vi "Teleop.vi"(10 "Match Info":T1={"Autonomous Elapsed Seconds"=0.0, "TeleOp Elapsed Seconds"=0.0, "Disabled Elapsed Seconds"=0.0, "Visited Autonomous"=FALSE, "Visited TeleOp"=FALSE, "Visited Disabled"=FALSE, "Autonomous Settings"={"Autonomous Style"=enum."Independent", "VI Refnum"=refnum}}, 11 "Call Context":T2) -> ()   [LabVIEW 2016]
doc: "This VI is called for each TeleOp packet received from the DS where the robot is not disabled. It is often used to read from the joysticks and update I/O or to update setpoints for timed control loops. It should complete and return within 20 milliseconds or it may miss DS packets."
uses:
  <vilib>/Rock Robotics/WPI/DriverStation/WPI_DriverStationDerivedRobotMode.ctl
  <vilib>/Rock Robotics/WPI/DriverStation/WPI_DriverStationMatch Info.ctl
  <vilib>/Rock Robotics/WPI/Solenoid/WPI_SolenoidValue.ctl
  <vilib>/Rock Robotics/WPI/Utilities/WPI_GetSetVariantRefNum.vi
  <vilib>/Rock Robotics/Network Tables/NT Read Boolean.vi
  <vilib>/Rock Robotics/Network Tables/NT Read Number.vi
  <vilib>/Rock Robotics/WPI/Solenoid/WPI_SolenoidSetEnum.vi
panel:
  in  "Compresseur Limit Time":bool
  in  "Reset":bool
  out "Droit":dbl
  out "Gauche":dbl
  in  "Quand arreter compresseur":dbl
  out "Teleop Time Elipsed":dbl
  out "Sample Slider 0":dbl(slide) scale=0.0..5.0
  out "Sample Boolean 1":bool
  out "Sample Boolean 0":bool
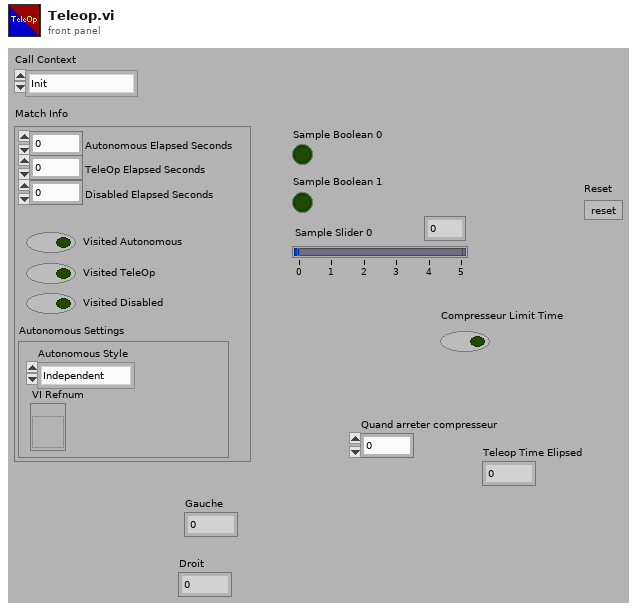
[diagram p1: front panel]
types:
  T1 = typedef "WPI_DriverStationMatch Info.ctl" = cluster{"Autonomous Elapsed Seconds":dbl, "TeleOp Elapsed Seconds":dbl, "Disabled Elapsed Seconds":dbl, "Visited Autonomous":bool, "Visited TeleOp":bool, "Visited Disabled":bool, "Autonomous Settings":cluster{"Autonomous Style":enum16{"Iterative", "Independent"}, "VI Refnum":refnum<vi>}}
  T2 = typedef "WPI_DriverStationDerivedRobotMode.ctl" = enum16{"Init", "Execute", "Stop"}
  T3 = typedef "WPI_JoystickDevRef.ctl" = cluster{"Device":T4}
  T4 = typedef "WPI_JoystickDeviceEnum.ctl" = enum16{"USB 0", "USB 1", "USB 2", "USB 3", "USB 4", "USB 5"}
  T5 = typedef "WPI_EncoderDevRef.ctl" = cluster{"DevStatus":errorcluster, "EncoderIndex":T6, "CounterIndex":T7, "DistancePerCount":dbl, "Decoding Type":T8}
  T6 = typedef "FPGA_EncoderIdx.ctl" = enum8{"Enc 0", "Enc 1", "Enc 2", "Enc 3", "Enc 4", "Enc 5", "Enc 6", "Enc 7", "Invalid"}
  T7 = typedef "FPGA_CounterCtrSystemIndex.ctl" = enum8{"Ctr 0", "Ctr 1", "Ctr 2", "Ctr 3", "Ctr 4", "Ctr 5", "Ctr 6", "Ctr 7", "Invalid"}
  T8 = typedef "WPI_EncoderType.ctl" = enum16{"1x", "2x", "4x"}
  T9 = cluster{"Axes[0]":dbl, "Axes[1]":dbl, "Axes[2]":dbl, "Axes[3]":dbl, "Axes[4]":dbl, "Axes[5]":dbl, "Axes[6]":dbl, "Axes[7]":dbl, "Axes[8]":dbl}
  T10 = cluster{"Buttons[0]":bool, "Buttons[1]":bool, "Buttons[2]":bool, "Buttons[3]":bool, "Buttons[4]":bool, "Buttons[5]":bool, "Buttons[6]":bool, "Buttons[7]":bool, "Buttons[8]":bool}
  T11 = typedef "WPI_RobotDriveDevRef.ctl" = cluster{"DevStatus":errorcluster, "Motors[]":T12[], "Square Inputs":bool, "Max Output":dbl}
  T12 = typedef "WPI_MotorControlDeviceRef.ctl" = cluster{"DeviceStatus":errorcluster, "Type":T13, "PWM":cluster{"PWM Channel":T14, "DeadBand":T15}, "CAN":cluster{"Device Number":u8, "SetOutput VI Ref":variant, "GetOutput VI Ref":variant, "Enable VI Ref":variant, "Disable VI Ref":variant, "Data":variant}, "Invert":bool}
  T13 = typedef "WPI_MotorControlType.ctl" = enum16{"PWM", "CAN"}
  T14 = typedef "FPGA_DIOPWMChannel.ctl" = enum8{"PWM 0", "PWM 1", "PWM 2", "PWM 3", "PWM 4", "PWM 5", "PWM 6", "PWM 7", "PWM 8", "PWM 9", "PWM MXP 0", "PWM MXP 1", "PWM MXP 2", "PWM MXP 3", "PWM MXP 4", "PWM MXP 5", "PWM MXP 6", "PWM MXP 7", "PWM MXP 8", "PWM MXP 9", "Invalid"}
  T15 = typedef "WPI_PWMDeadband.ctl" = cluster{"Name":string, "maxPositivePwm":i32, "minPositivePwm":i32, "centerPwm":i32, "maxNegativePwm":i32, "minNegativePwm":i32, "angularRange":u16}
  T16 = typedef "WPI_SolenoidValue.ctl" = enum16{"Off", "On", "Forward", "Reverse"}
  T17 = typedef "WPI_SolenoidDevRef.ctl" = cluster{"DevStatus":errorcluster, "Pneumatics Control Module":u8, "Forward Solenoid Channel":T18, "Reverse Solenoid Channel":T18}
  T18 = typedef "WPI_SolenoidChannel.ctl" = enum8{"Solenoid 0", "Solenoid 1", "Solenoid 2", "Solenoid 3", "Solenoid 4", "Solenoid 5", "Solenoid 6", "Solenoid 7", "Invalid"}
  T19 = typedef "WPI_CompressorDevRef.ctl" = cluster{"DevStatus":errorcluster, "Pneumatics Control Module":u8}
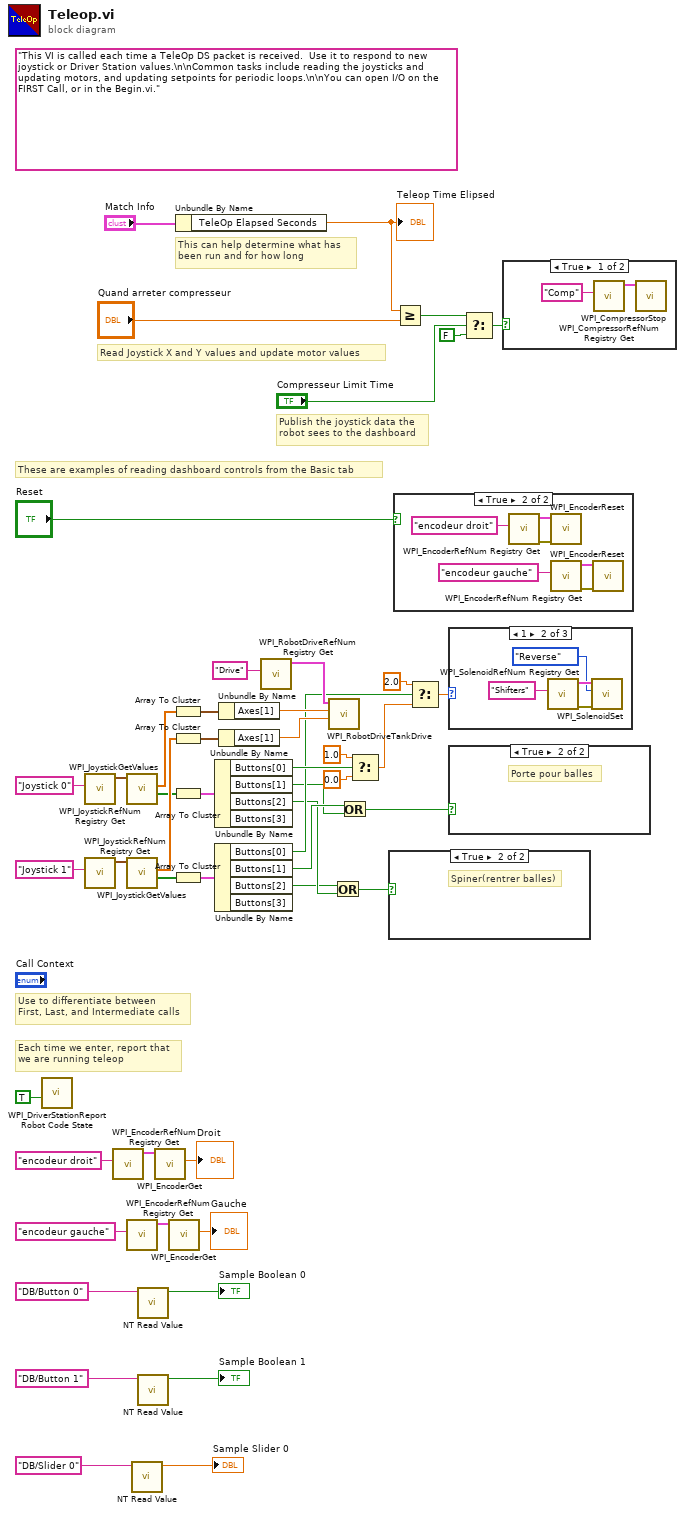
[diagram p0: block diagram]
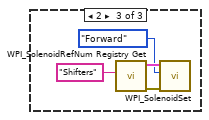
[diagram p7: hidden frame]
diagram:
  (unwired) "This VI is called each time a TeleOp DS packet is received.  Use it to respond to new joystick or Driver Station values.\n\nCommon tasks include reading the joysticks and updating motors, and updating setpoints for periodic loops.\n\nYou can open I/O on the FIRST Call, or in the Begin.vi."
  # "These are examples of reading dashboard controls from the Basic tab"
  # "Publish the joystick data the\nrobot sees to the dashboard"
  # "Each time we enter, report that\nwe are running teleop"
  # "Use to differentiate between\nFirst, Last, and Intermediate calls"
  # "This can help determine what has\nbeen run and for how long"
  # "Read Joystick X and Y values and update motor values"
  n1 = call <vilib>:"WPI_DriverStationReport Robot Code State.vi"("TeleOp"=TRUE ("Autonomous")) -> ()  [unwired: 10 in, 1 out]
  n2 = call <vilib>:"WPI_JoystickRefNum Registry Get.vi"("refnum name"="Joystick 0") -> ("JoystickDevRef"=w48:T3)  [unwired: 1 in, 9 out]
  n3 = call <vilib>:"WPI_JoystickRefNum Registry Get.vi"("refnum name"="Joystick 1") -> ("JoystickDevRef"=w36:T3)  [unwired: 1 in, 9 out]
  n4 = call <vilib>:"WPI_EncoderRefNum Registry Get.vi"("refnum name"="encodeur droit") -> ("EncoderDevRef"=w16:T5)  [unwired: 9 in, 1 out]
  n5 = call <vilib>:"WPI_JoystickGetValues.vi"("JoystickDevRef"=w48) -> ("Buttons"=w27:bool[], "Axes"=w39:dbl[])  [unwired: 6 in, 3 out]
  n6 = call <vilib>:"WPI_JoystickGetValues.vi"("JoystickDevRef"=w36) -> ("Buttons"=w30:bool[], "Axes"=w35:dbl[])  [unwired: 6 in, 3 out]
  n7 = call <vilib>:"WPI_EncoderRefNum Registry Get.vi"("refnum name"="encodeur gauche") -> ("EncoderDevRef"=w17:T5)  [unwired: 9 in, 1 out]
  n8 = call-poly <vilib>:"NT Read Value.vi"("Name"="DB/Slider 0" ("refnum name")) -> ("Numeric"=→"Sample Slider 0":dbl)  [unwired: 9 in, 1 out]
  n9 = call-poly <vilib>:"NT Read Value.vi"("Name"="DB/Button 0" ("refnum name")) -> ("Boolean"=→"Sample Boolean 0":bool)  [unwired: 9 in, 1 out]
  n10 = call-poly <vilib>:"NT Read Value.vi"("Name"="DB/Button 1" ("refnum name")) -> ("Boolean"=→"Sample Boolean 1":bool)  [unwired: 9 in, 1 out]
  n11 = call <vilib>:"WPI_EncoderGet.vi"("EncoderDevRef"=w16) -> ("Distance"=→"Droit":dbl)  [unwired: 5 in, 5 out]
  n12 = call <vilib>:"WPI_EncoderGet.vi"("EncoderDevRef"=w17) -> ("Distance"=→"Gauche":dbl)  [unwired: 5 in, 5 out]
  n13 = Array To Cluster(array=w39) -> (cluster=w38:T9)
  n14 = Array To Cluster(array=w35) -> (cluster=w34:T9)
  n15 = Array To Cluster(array=w27) -> (cluster=w28:T10)
  n16 = Array To Cluster(array=w30) -> (cluster=w29:T10)
  n17 = Unbundle By Name("Match Info") -> ("TeleOp Elapsed Seconds"=w18:dbl)
  "Teleop Time Elipsed" <- w18
  n18 = Unbundle By Name(w28) -> ("Buttons[0]"=w24:bool, "Buttons[1]"=w9:bool, "Buttons[2]"=w8:bool)  [unwired: 1 out]
  n19 = Unbundle By Name(w29) -> ("Buttons[0]"=w22:bool, "Buttons[1]"=w10:bool, "Buttons[2]"=w7:bool)  [unwired: 1 out]
  n20 = Unbundle By Name(w38) -> ("Axes[1]"=w32:dbl)
  n21 = Unbundle By Name(w34) -> ("Axes[1]"=w31:dbl)
  n22 = call <vilib>:"WPI_RobotDriveRefNum Registry Get.vi"("refnum name"="Drive") -> ("RobotDriveDevRef"=w40:T11)  [unwired: 9 in, 1 out]
  n23 = call <vilib>:"WPI_RobotDriveTankDrive.vi"("Right axis value"=w31, "Left axis value"=w32, "RobotDriveDevRef"=w40) -> ()  [unwired: 6 in, 3 out]
  n24 = Or(x=w7, y=w8) -> (x .or. y?=w6:bool)
  n25 = Or(x=w10, y=w9) -> (x .or. y?=w5:bool)
  n26 = Select(t=1.0, s=w24, f=0.0) -> (s? t:f=w26:dbl)
  n27 = case shown="True" w6 {
    frame False {
    }
    frame True {
      # "Spiner(rentrer balles)"
    }
  }
  n28 = case shown="True" "Reset" {
    frame False {
    }
    frame True {
      n29 = call <vilib>:"WPI_EncoderRefNum Registry Get.vi"("refnum name"="encodeur droit") -> ("error out"=w53:errorcluster, "EncoderDevRef"=w54:T5)  [unwired: 9 in]
      n30 = call <vilib>:"WPI_EncoderReset.vi"("error in (no error)"=w53, "EncoderDevRef"=w54) -> ()  [unwired: 8 in, 2 out]
      n31 = call <vilib>:"WPI_EncoderRefNum Registry Get.vi"("refnum name"="encodeur gauche") -> ("error out"=w52:errorcluster, "EncoderDevRef"=w51:T5)  [unwired: 9 in]
      n32 = call <vilib>:"WPI_EncoderReset.vi"("error in (no error)"=w52, "EncoderDevRef"=w51) -> ()  [unwired: 8 in, 2 out]
    }
  }
  n33 = Greater Or Equal?(x=w18, y="Quand arreter compresseur") -> (x >= y?=w4:bool)
  n34 = Select(t=2.0, s=w22, f=w26) -> (s? t:f=w21:dbl)
  n35 = case shown="1" w21 {
    frame 0, Default {
    }
    frame 1 {
      n36 = call <vilib>:"WPI_SolenoidRefNum Registry Get.vi"("refnum name"="Shifters") -> ("error out"=w59:errorcluster, "SolenoidDevRef"=w58:T17)  [unwired: 9 in]
      n37 = call-poly <vilib>:"WPI_SolenoidSet.vi"("error in (no error)"=w59, "Value"=WPI_SolenoidValue."Reverse", "SolenoidDevRef"=w58) -> ()  [unwired: 7 in, 2 out]
    }
    frame 2 {
      n38 = call <vilib>:"WPI_SolenoidRefNum Registry Get.vi"("refnum name"="Shifters") -> ("error out"=w63:errorcluster, "SolenoidDevRef"=w62:T17)  [unwired: 9 in]
      n39 = call-poly <vilib>:"WPI_SolenoidSet.vi"("error in (no error)"=w63, "Value"=WPI_SolenoidValue."Forward", "SolenoidDevRef"=w62) -> ()  [unwired: 7 in, 2 out]
    }
  }
  n40 = case shown="True" w5 {
    frame False {
    }
    frame True {
      # "Porte pour balles"
    }
  }
  n41 = Select(t=w4, s="Compresseur Limit Time", f=FALSE) -> (s? t:f=w1:bool)
  n42 = case shown="True" w1 {
    frame True {
      n43 = call <vilib>:"WPI_CompressorRefNum Registry Get.vi"("refnum name"="Comp") -> ("CompressorDevRef"=w66:T19)  [unwired: 9 in, 1 out]
      n44 = call <vilib>:"WPI_CompressorStop.vi"("CompressorDevRef"=w66) -> ()  [unwired: 9 in, 2 out]
    }
    frame False {
    }
  }
